vi "setParameters.vi"(10 "Parameters":T1, 11 "ManipulateM1M3Command in":refnum<class "ManipulateM1M3Command.lvclass">) -> (3 "ManipulateM1M3Command out":refnum<class "ManipulateM1M3Command.lvclass">)   [LabVIEW 2016, in "ManipulateM1M3Command.lvclass"]
uses:
  ManipulateM1M3Command.lvclass
  DataTypes/Topics/CommandManipulateM1M3.ctl
  DataTypes/Topics/Parts/CommandId.ctl
  ManipulateM1M3Command.lvclass/ManipulateM1M3Command.ctl
  DataTypes/Topics/M1M3SupportTopics.lvlib
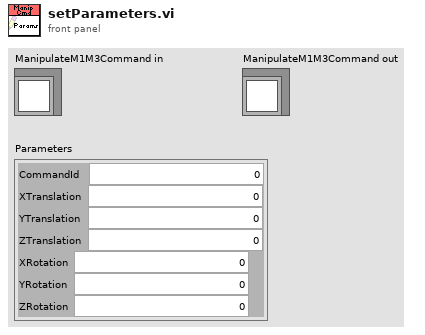
[diagram p1: front panel]
types:
  T1 = typedef "M1M3SupportTopics.lvlib/CommandManipulateM1M3.ctl" = cluster{"CommandId":T2, "XTranslation":dbl, "YTranslation":dbl, "ZTranslation":dbl, "XRotation":dbl, "YRotation":dbl, "ZRotation":dbl}
  T2 = typedef "M1M3SupportTopics.lvlib/CommandId.ctl" = i32
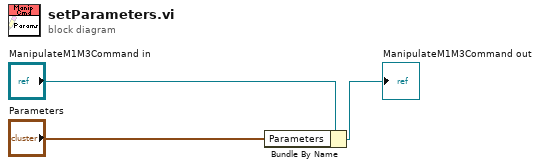
[diagram p0: block diagram]
diagram:
  n1 = Bundle By Name(cluster="ManipulateM1M3Command in", "Parameters"="Parameters") -> (→"ManipulateM1M3Command out":refnum<class "ManipulateM1M3Command.lvclass">)
